vi "Create Cubes.vi"(4 "Y Dimension":i32, 5 "Width":sgl, 6 "X Dimension":i32, 7 "Bar Mode":enum16{"Detach", "Group", "Stack"}(ring), 9 "Difference":sgl, 11 "Bar Info In":cluster{"X":sgl, "Y":sgl, "Z":sgl}[](array[cluster])) -> (3 "Vertex Array Out":cluster{"X":sgl, "Y":sgl, "Z":sgl}[](array[cluster]))   [LabVIEW 2017, in "3D Bar.lvclass"]
uses:
  <vilib>/Math Plots/3D Math Plots/3D Bar/3D Bar/3D Bar.lvclass
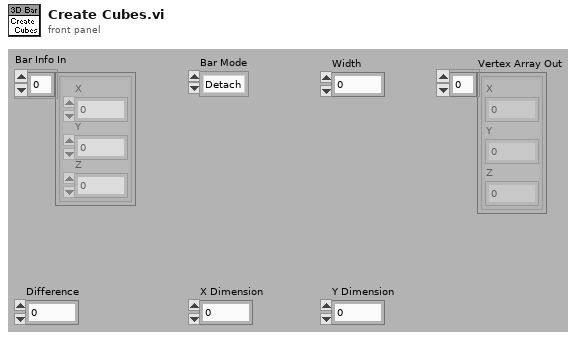
[diagram p1: front panel]
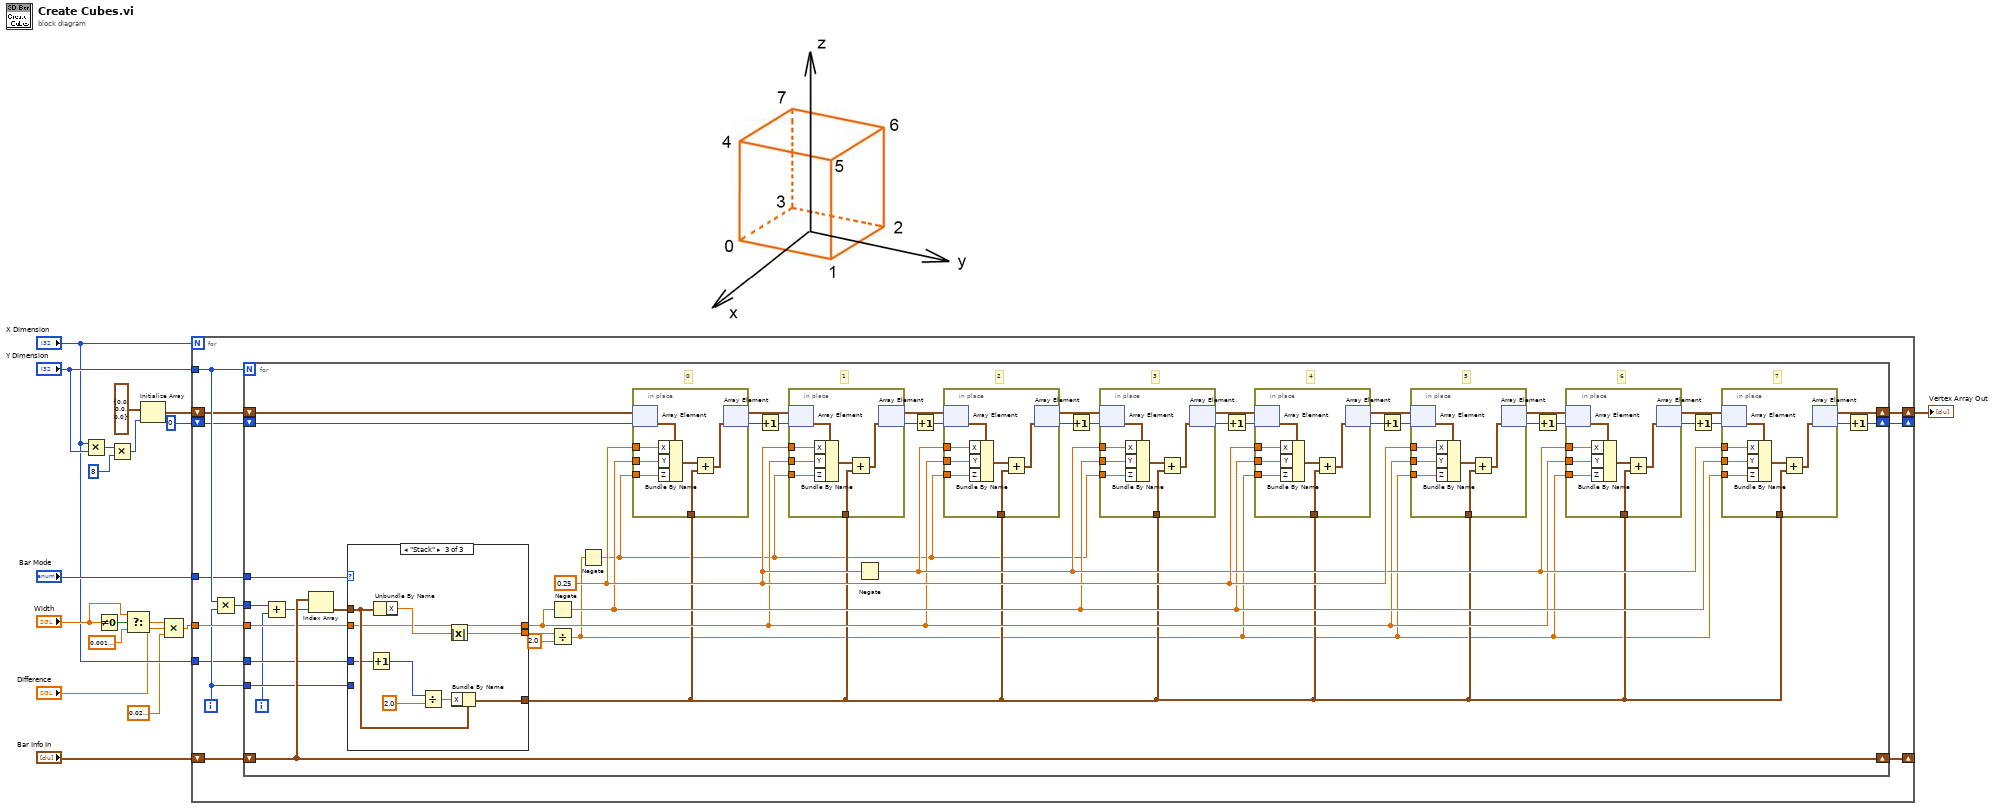
[diagram p0: block diagram]
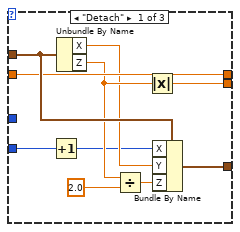
[diagram p2: hidden frame]
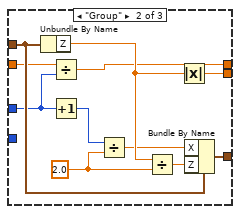
[diagram p3: hidden frame]
diagram:
  n1 = Multiply(x="X Dimension", y="Y Dimension") -> (x*y=w6:i32)
  n2 = Not Equal To 0?(x="Width") -> (x != 0?=w15:bool)
  n3 = Multiply(x=w6, y=8 ("value")) -> (x*y=w7:i32)
  n4 = Select(t="Width", s=w15, f=sgl 0.001) -> (s? t:f=w12:sgl)
  n5 = Initialize Array(cluster{"X":sgl, "Y":sgl, "Z":sgl} {"X"=0.0, "Y"=0.0, "Z"=0.0} ("3D Point"), w7) -> (w10:cluster{"X":sgl, "Y":sgl, "Z":sgl}[])
  n6 = Compound Arithmetic op=MULTIPLY(w12, "Difference", sgl 0.03 ("value")) -> (w18:sgl)
  n7 = for {
    N: "X Dimension" -> [_]
    tunnel: w18 -> [w28]
    tunnel: "Y Dimension" -> [w27]
    shift-right: [w29] -> _
    shift-left: "Bar Info In" -> [w30]
    tunnel: "Bar Mode" -> [w25]
    tunnel: "X Dimension" -> [w23]
    shift-right: [w20] -> w3
    shift-left: w10 -> [w22]
    shift-right: [w19] -> _
    shift-left: 0 -> [w21]
    i -> [w24]
    n8 = Multiply(x=w27, y=w24) -> (x*y=w26:i32)
    n9 = for {
      N: w27 -> [_]
      tunnel: w28 -> [w69]
      shift-right: [w72] -> w29
      shift-left: w30 -> [w72]
      tunnel: w26 -> [w73]
      tunnel: w25 -> [w70]
      tunnel: w24 -> [w68]
      tunnel: w23 -> [w67]
      shift-right: [w55] -> w20
      shift-left: w22 -> [w65]
      shift-right: [w41] -> w19
      shift-left: w21 -> [w35]
      i -> [w66]
      w40 = sgl 0.25 ("Length X")
      # "7"
      # "6"
      # "5"
      # "4"
      # "3"
      # "2"
      # "1"
      # "0"
      n10 = Add(x=w73, y=w66) -> (x+y=w71:i32)
      n11 = Index Array(array=w72, index=w71) -> (element=w74:cluster{"X":sgl, "Y":sgl, "Z":sgl})
      n12 = case shown="\"Stack\"" w70 {
        tunnel: [w140 w148 w158] -> w36
        tunnel: [w131 w141 w152] -> w34
        tunnel: w74 -> [w137 w150 w160]
        tunnel: w69 -> [w136 w147 w157]
        tunnel: [w136 w146 w157] -> w37
        tunnel: w68 -> [w133 _ _]
        tunnel: w67 -> [_ w144 w153]
        frame "Detach" {
          n13 = Increment(x=w133) -> (x+1=w132:i32)
          n14 = Unbundle By Name(w137) -> ("X"=w134:sgl, "Z"=w135:sgl)
          n15 = Divide(x=w135, y=sgl 2.0) -> (x/y=w139:sgl)
          n16 = Absolute Value(x=w135) -> (abs(x)=w131:sgl)
          n17 = Bundle By Name(cluster=w137, "X"=w132, "Y"=w134, "Z"=w139) -> (w140:cluster{"X":sgl, "Y":sgl, "Z":sgl})
        }
        frame "Group" {
          w142 = sgl 2.0 ("y")
          n18 = Unbundle By Name(w150) -> ("Z"=w149:sgl)
          n19 = Divide(x=w147, y=w144) -> (x/y=w146:sgl)
          n20 = Increment(x=w144) -> (x+1=w145:i32)
          n21 = Divide(x=w145, y=w142) -> (x/y=w143:sgl)
          n22 = Divide(x=w149, y=w142) -> (x/y=w151:sgl)
          n23 = Absolute Value(x=w149) -> (abs(x)=w141:sgl)
          n24 = Bundle By Name(cluster=w150, "X"=w143, "Z"=w151) -> (w148:cluster{"X":sgl, "Y":sgl, "Z":sgl})
        }
        frame "Stack" {
          n25 = Increment(x=w153) -> (x+1=w156:i32)
          n26 = Unbundle By Name(w160) -> ("X"=w159:sgl)
          n27 = Divide(x=w156, y=sgl 2.0 ("X")) -> (x/y=w154:sgl)
          n28 = Absolute Value(x=w159) -> (abs(x)=w152:sgl)
          n29 = Bundle By Name(cluster=w160, "X"=w154) -> (w158:cluster{"X":sgl, "Y":sgl, "Z":sgl})
        }
      }
      n30 = Negate(x=w37) -> (-x=w38:sgl)
      n31 = Divide(x=w34, y=sgl 2.0) -> (x/y=w31:sgl)
      n32 = Negate(x=w31) -> (-x=w32:sgl)
      n33 = in-place {
        in-place-border: w40 -> [w129]
        in-place-border: w38 -> [w128]
        in-place-border: w36 -> [w125]
        in-place-border: w32 -> [w124]
        n34 = in-place-array #1(w65, w35) -> (w130:cluster{"X":sgl, "Y":sgl, "Z":sgl})
        n35 = Bundle By Name(cluster=w130, "X"=w129, "Y"=w128, "Z"=w124) -> (w127:cluster{"X":sgl, "Y":sgl, "Z":sgl})
        n36 = Add(x=w127, y=w125) -> (x+y=w126:cluster{"X":sgl, "Y":sgl, "Z":sgl})
        n37 = in-place-array #1(w126) -> (w64:cluster{"X":sgl, "Y":sgl, "Z":sgl}[], w63:i32)
      }
      n38 = Increment(x=w63) -> (x+1=w62:i32)
      n39 = in-place {
        in-place-border: w40 -> [w122]
        in-place-border: w37 -> [w121]
        in-place-border: w32 -> [w120]
        in-place-border: w36 -> [w117]
        n40 = in-place-array #2(w64, w62) -> (w123:cluster{"X":sgl, "Y":sgl, "Z":sgl})
        n41 = Bundle By Name(cluster=w123, "X"=w122, "Y"=w121, "Z"=w120) -> (w119:cluster{"X":sgl, "Y":sgl, "Z":sgl})
        n42 = Add(x=w119, y=w117) -> (x+y=w118:cluster{"X":sgl, "Y":sgl, "Z":sgl})
        n43 = in-place-array #2(w118) -> (w54:cluster{"X":sgl, "Y":sgl, "Z":sgl}[], w48:i32)
      }
      n44 = Negate(x=w40) -> (-x=w39:sgl)
      n45 = Increment(x=w48) -> (x+1=w61:i32)
      n46 = in-place {
        in-place-border: w39 -> [w115]
        in-place-border: w37 -> [w114]
        in-place-border: w32 -> [w113]
        in-place-border: w36 -> [w111]
        n47 = in-place-array #3(w54, w61) -> (w116:cluster{"X":sgl, "Y":sgl, "Z":sgl})
        n48 = Bundle By Name(cluster=w116, "X"=w115, "Y"=w114, "Z"=w113) -> (w112:cluster{"X":sgl, "Y":sgl, "Z":sgl})
        n49 = Add(x=w112, y=w111) -> (x+y=w110:cluster{"X":sgl, "Y":sgl, "Z":sgl})
        n50 = in-place-array #3(w110) -> (w53:cluster{"X":sgl, "Y":sgl, "Z":sgl}[], w47:i32)
      }
      n51 = Increment(x=w47) -> (x+1=w60:i32)
      n52 = in-place {
        in-place-border: w39 -> [w108]
        in-place-border: w38 -> [w107]
        in-place-border: w32 -> [w106]
        in-place-border: w36 -> [w104]
        n53 = in-place-array #4(w53, w60) -> (w109:cluster{"X":sgl, "Y":sgl, "Z":sgl})
        n54 = Bundle By Name(cluster=w109, "X"=w108, "Y"=w107, "Z"=w106) -> (w105:cluster{"X":sgl, "Y":sgl, "Z":sgl})
        n55 = Add(x=w105, y=w104) -> (x+y=w103:cluster{"X":sgl, "Y":sgl, "Z":sgl})
        n56 = in-place-array #4(w103) -> (w52:cluster{"X":sgl, "Y":sgl, "Z":sgl}[], w46:i32)
      }
      n57 = Increment(x=w46) -> (x+1=w59:i32)
      n58 = in-place {
        in-place-border: w40 -> [w101]
        in-place-border: w38 -> [w100]
        in-place-border: w31 -> [w99]
        in-place-border: w36 -> [w97]
        n59 = in-place-array #5(w52, w59) -> (w102:cluster{"X":sgl, "Y":sgl, "Z":sgl})
        n60 = Bundle By Name(cluster=w102, "X"=w101, "Y"=w100, "Z"=w99) -> (w98:cluster{"X":sgl, "Y":sgl, "Z":sgl})
        n61 = Add(x=w98, y=w97) -> (x+y=w96:cluster{"X":sgl, "Y":sgl, "Z":sgl})
        n62 = in-place-array #5(w96) -> (w51:cluster{"X":sgl, "Y":sgl, "Z":sgl}[], w45:i32)
      }
      n63 = Increment(x=w45) -> (x+1=w58:i32)
      n64 = in-place {
        in-place-border: w40 -> [w94]
        in-place-border: w37 -> [w93]
        in-place-border: w31 -> [w92]
        in-place-border: w36 -> [w90]
        n65 = in-place-array #6(w51, w58) -> (w95:cluster{"X":sgl, "Y":sgl, "Z":sgl})
        n66 = Bundle By Name(cluster=w95, "X"=w94, "Y"=w93, "Z"=w92) -> (w91:cluster{"X":sgl, "Y":sgl, "Z":sgl})
        n67 = Add(x=w91, y=w90) -> (x+y=w89:cluster{"X":sgl, "Y":sgl, "Z":sgl})
        n68 = in-place-array #6(w89) -> (w50:cluster{"X":sgl, "Y":sgl, "Z":sgl}[], w44:i32)
      }
      n69 = Increment(x=w44) -> (x+1=w57:i32)
      n70 = in-place {
        in-place-border: w39 -> [w87]
        in-place-border: w37 -> [w86]
        in-place-border: w31 -> [w85]
        in-place-border: w36 -> [w82]
        n71 = in-place-array #7(w50, w57) -> (w88:cluster{"X":sgl, "Y":sgl, "Z":sgl})
        n72 = Bundle By Name(cluster=w88, "X"=w87, "Y"=w86, "Z"=w85) -> (w84:cluster{"X":sgl, "Y":sgl, "Z":sgl})
        n73 = Add(x=w84, y=w82) -> (x+y=w83:cluster{"X":sgl, "Y":sgl, "Z":sgl})
        n74 = in-place-array #7(w83) -> (w49:cluster{"X":sgl, "Y":sgl, "Z":sgl}[], w43:i32)
      }
      n75 = Increment(x=w43) -> (x+1=w56:i32)
      n76 = in-place {
        in-place-border: w39 -> [w80]
        in-place-border: w38 -> [w79]
        in-place-border: w31 -> [w78]
        in-place-border: w36 -> [w76]
        n77 = in-place-array #8(w49, w56) -> (w81:cluster{"X":sgl, "Y":sgl, "Z":sgl})
        n78 = Bundle By Name(cluster=w81, "X"=w80, "Y"=w79, "Z"=w78) -> (w77:cluster{"X":sgl, "Y":sgl, "Z":sgl})
        n79 = Add(x=w77, y=w76) -> (x+y=w75:cluster{"X":sgl, "Y":sgl, "Z":sgl})
        n80 = in-place-array #8(w75) -> (w55:cluster{"X":sgl, "Y":sgl, "Z":sgl}[], w42:i32)
      }
      n81 = Increment(x=w42) -> (x+1=w41:i32)
    }
  }
  "Vertex Array Out" <- w3
